vi "STAGE+mono+counter_edit16.vi"() -> ()   [LabVIEW 2017]
panel:
  out "XY Graph 2":cluster{dbl[], dbl[]}[](graph)
  out "XY Graph":cluster{dbl[], dbl[]}(graph)
  out "PROGRESS":u8(slide) max=10 step=10 scale=0.0..1.0
  in  "?":enum32{"DELAY", "COUNTER", "MONO", "PLOT"}(tab)
  out "Final time [ps]":dbl
  out "Current time [ps]":dbl
  out "Initial time [ps]":dbl
  in  "Set this as t0":bool
  in  "Axis":i32=1
  in  "Motor ON":bool
  in  "Motor OFF":bool
  out "Current Position [mm]":dbl
  out "Final Position [mm]":dbl
  in  "Data Points":i32=100
  out "Current Point":i32
  in  "Step Size [um]":i32=10
  in  "Target [mm]":dbl format="%.3f"
  in  "Move":bool
  out "Initial position [mm]":dbl
  in  "GPIB address":string="23"
  in  "Count Mode":u16(ring) items=["A,B for Preset T", "A-B for Preset T", "A+B for Preset T", "A for Preset B"]
  in  "Trigger mode":u16(ring) items=["10 MHz"=0, "Input 2"=2, "Input T"=3]
  in  "Channel A Input":u16(ring)=1 items=["10 MHz", "Input 1"]
  in  "Channel B Input":u16(ring)=2 items=["Input 1"=1, "Input 2"=2]
  in  "Number of Measurements\n to take at one point/ Number of Periods":u16=1 min=1 max=2000 step=1
  in  "Time between measurements\n at one point (s)/Dwell Time":dbl=0.002 min=0.002 max=60.0 step=0.001
  in  "gate mode (CW:0)":i16(slide) scale=0.0..2.0 scale format="%.2f"
  out "Counts":i32
  in  "Integrating time \nin 10^-7 sec":dbl=10000000.0
  in  "Discriminator Level (mV)":dbl min=-300.0 max=300.0 step=0.2
  in  "Discriminator Slope":bool
  in  "Channel":i16 min=0 max=2 step=1
  out "Grating #":dbl
  out "Blaze angle":dbl
  out "Grooves/mm":dbl
  out "Mono port":T1(ring)
  out "Time delay":u32=450000 min=1
  in  "Step size":dbl=10.0 min=0.0
  in  "Scan to":i32=4000
  in  "Scan from":i32=2600
  out "Current wavelength":dbl
  in  "?":bool
  in  "Array":dbl[](array[numeric])
  out "Numeric":i32
  out "Numeric 2":i32
  out "Timeout 2":bool
  in  "?":bool
  out "Timeout":bool
  in  "Collect Data!":bool
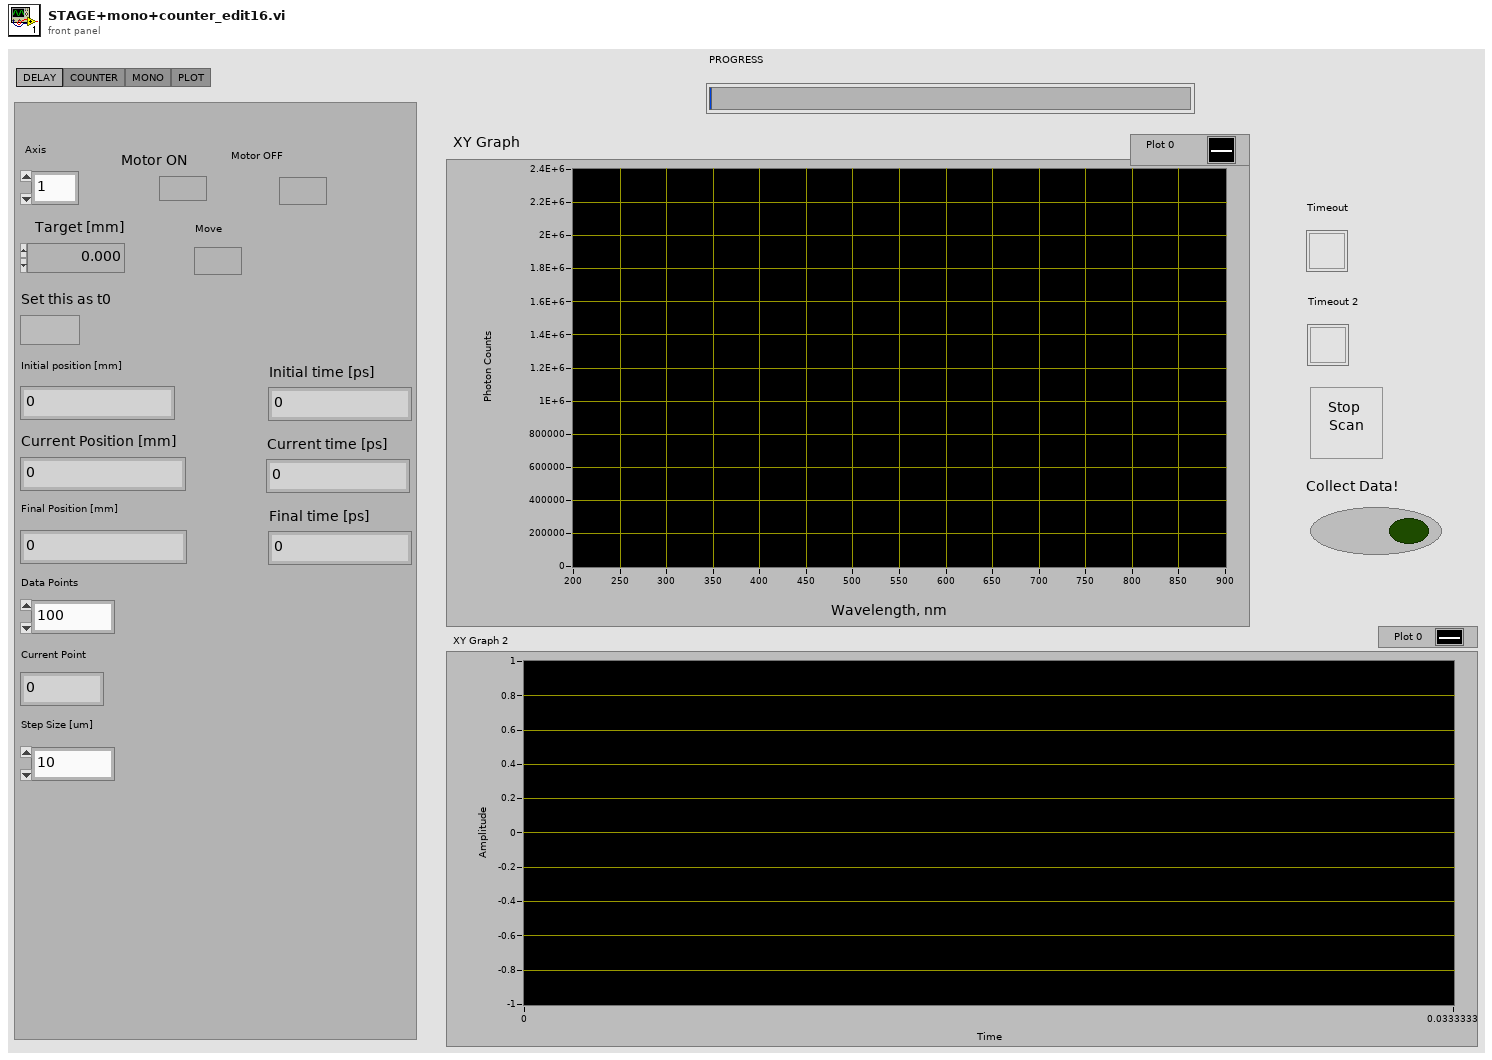
[diagram p1: front panel]
types:
  T1 = enum8{"COM 1", "COM 2", "COM 3", "COM 4", "COM 5", "COM 6", "COM 7", "COM 8", "COM 9"}
  T2 = cluster{"input XON/XOFF":bool, "input HW Handshake":bool, "input alt HW HShk":bool, "output XON/XOFF":bool, "output HW Handshake":bool, "output alt HW HShk":bool, "XOFF byte":u8, "XON byte":u8, "parity error byte":u16}
  T3 = enum16{"no parity", "odd parity", "even parity", "mark parity", "space parity"}
  T4 = cluster{"Y[0]":dbl, "Y[1]":dbl, "Y[2]":dbl, "Y[3]":dbl, "Y[4]":dbl, "Y[5]":dbl, "Y[6]":dbl, "Y[7]":dbl, "Y[8]":dbl}
  T5 = typedef "NI_Matrix.lvlib/RealMatrix.ctl" = dbl[][]
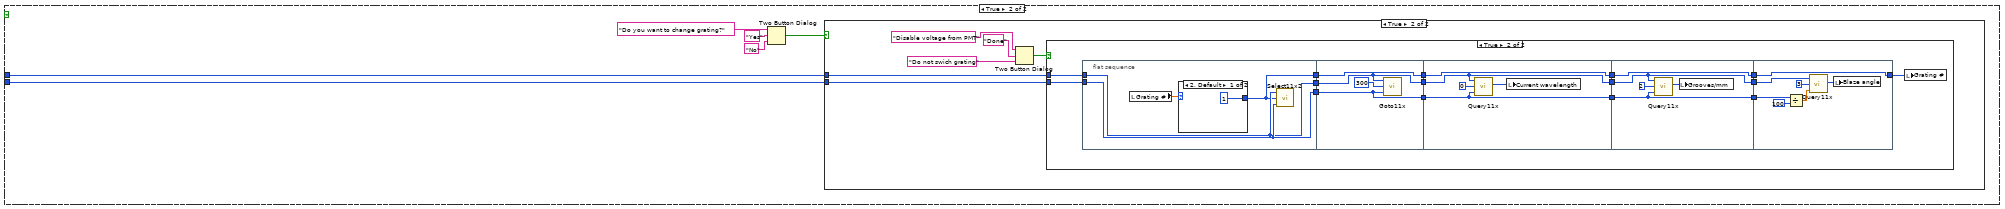
[diagram p2: hidden frame]
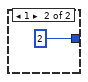
[diagram p5: hidden frame]
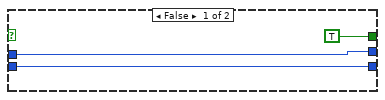
[diagram p6: hidden frame]
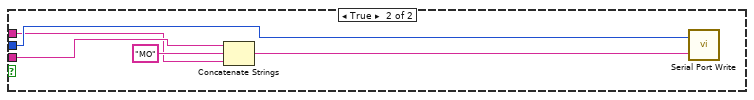
[diagram p7: hidden frame]
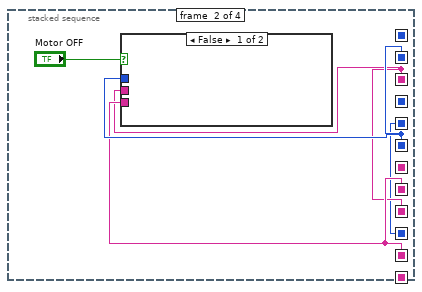
[diagram p8: hidden frame]
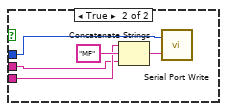
[diagram p9: hidden frame]
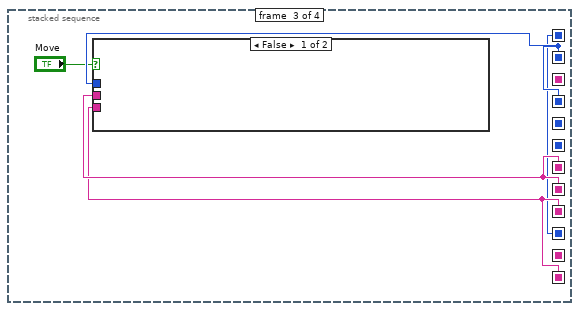
[diagram p10: hidden frame]
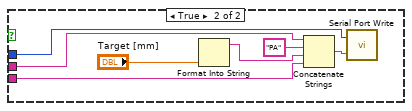
[diagram p11: hidden frame]
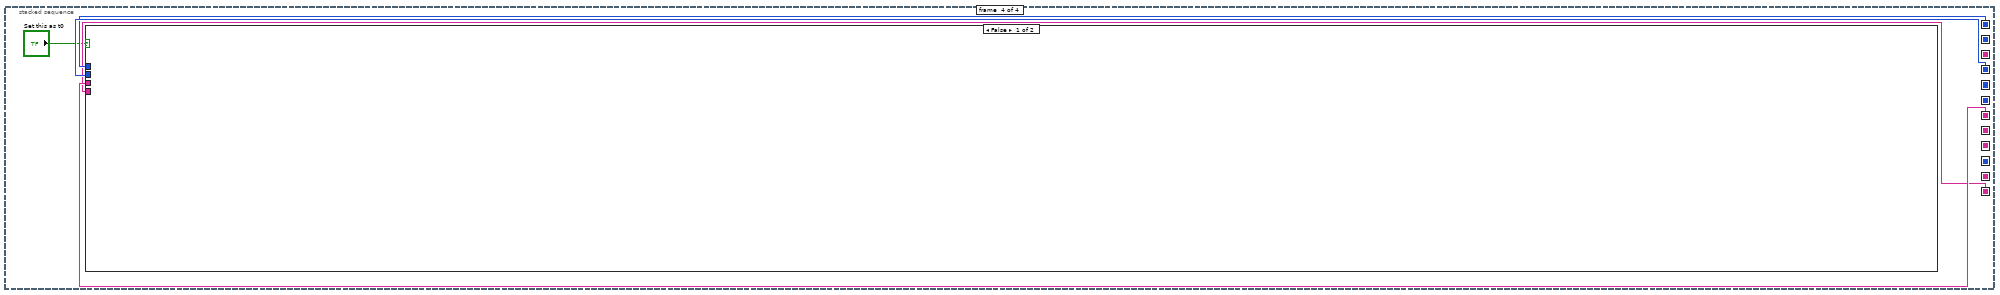
[diagram p12: hidden frame]
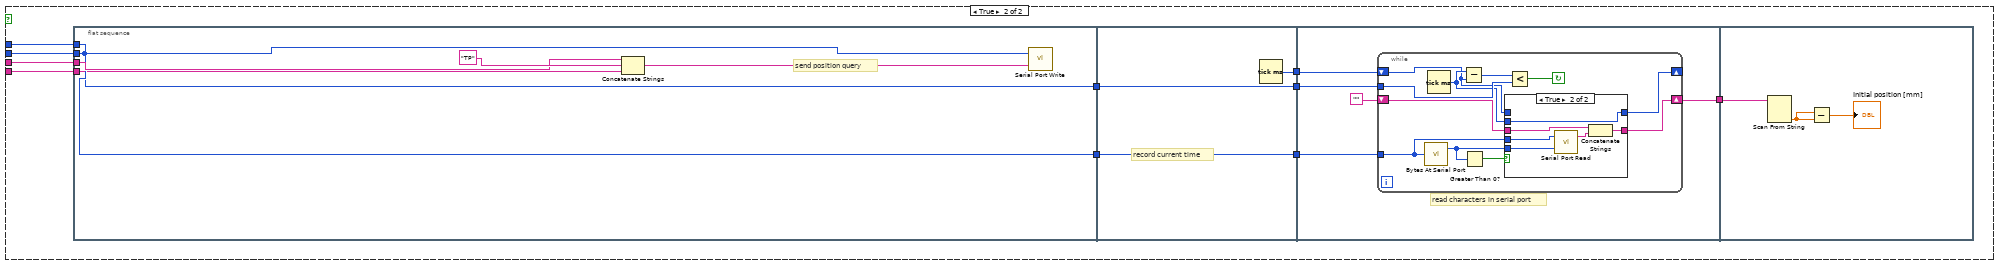
[diagram p13: hidden frame]
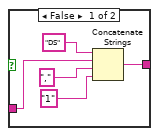
[diagram p15: hidden frame]
diagram:
  (unwired) FALSE
  w39 = u32 19200  # baud rate
  w38 = u16 8  # data bits
  w37 = enum16{"1 bit", "1.5 bits", "2 bits"}."1 bit"  # stop bits
  w41 = T3."no parity"  # parity
  w36 = 4  # 0=COM1 so n=COM(n+1)
  w40 = u16 1024  # buffer size
  n1 = flat-sequence {
    tunnel: ["Data Points"] -> w45
    tunnel: "Axis" -> [w67]
    tunnel: [w59] -> w44
    tunnel: [w67] -> w43
    tunnel: ["Step Size [um]"] -> w17
    tunnel: [w59] -> w16
    tunnel: ["Step Size [um]"] -> w15
    tunnel: ["Data Points"] -> w14
    tunnel: [w59] -> w13
    tunnel: [w58] -> w12
    tunnel: [w59] -> w10
    tunnel: [w58] -> w9
    tunnel: [w61] -> w8
    tunnel: [w51] -> w7
    tunnel: w45 -> [w151]
    tunnel: w44 -> [w150]
    tunnel: w43 -> [w149]
    tunnel: w36 -> [w145]
    tunnel: "GPIB address" -> [w144]
    tunnel: "GPIB address" -> [w143]
    tunnel: w17 -> [w131]
    tunnel: w16 -> [w129]
    tunnel: w15 -> [w128]
    tunnel: w14 -> [w126]
    tunnel: w13 -> [w121]
    tunnel: w12 -> [w120]
    tunnel: "Integrating time \nin 10^-7 sec" -> [w119]
    tunnel: w10 -> [w117]
    tunnel: w9 -> [w116]
    tunnel: w8 -> [w115]
    tunnel: w7 -> [w113]
    tunnel: w3 -> [w94]
    tunnel: w2 -> [w93]
    tunnel: w1 -> [w92]
    frame #0 {
      n2 = while {
        stop <- "Collect Data!" stop-if-true
        n3 = Multiply(x=1, y=1000) -> (x*y=w49:i32)
        n4 = Wait (ms)(milliseconds to wait=w49) -> ()  [unwired: 1 out]
      }
    }
    frame #1 {
      w52 = 1000000000000.0
      w57 = 1000
      w60 = 300000000
      w62 = 1000
      n5 = local read "Initial position [mm]"() -> (w59:dbl)
      n6 = Multiply(x="Step Size [um]", y="Data Points") -> (x*y=w66:i32)
      n7 = Divide(x=w66, y=w62) -> (x/y=w65:dbl)
      n8 = Divide(x="Step Size [um]", y=w62) -> (x/y=w61:dbl)
      n9 = Add(x=w59, y=w65) -> (x+y=w58:dbl)
      "Final Position [mm]" <- w58
      n10 = Divide(x=w59, y=w57) -> (x/y=w55:dbl)
      n11 = Divide(x=w58, y=w57) -> (x/y=w56:dbl)
      n12 = Divide(x=w55, y=w60) -> (x/y=w54:dbl)
      n13 = Divide(x=w56, y=w60) -> (x/y=w53:dbl)
      n14 = Multiply(x=w53, y=w52) -> (x*y=→"Final time [ps]":dbl)
      n15 = Multiply(x=w54, y=w52) -> (x*y=w51:dbl)
      "Initial time [ps]" <- w51
    }
    frame #2 {
      w74 = "\r\n"
      n16 = Increment(x=w126) -> (x+1=w127:i32)
      n17 = Divide(x=w131, y=1000.0) -> (x/y=w107:dbl)
      n18 = for {
        N: w127 -> [_]
        tunnel: w107 -> [w162]
        tunnel: w129 -> [w160]
        tunnel: [w153] -> w125 mode=indexing
        i -> [w161]
        # "distances"
        n19 = Multiply(x=w162, y=w161) -> (x*y=w159:dbl)
        n20 = Add(x=w160, y=w159) -> (x+y=w158:dbl)
        n21 = Divide(x=w158, y=1000) -> (x/y=w152:dbl)
        n22 = Divide(x=w152, y=300000000) -> (x/y=w155:dbl)
        n23 = Multiply(x=w155, y=1000000000000.0) -> (x*y=w153:dbl)
      }
      n24 = Multiply(x="Scan to", y=1) -> (x*y=w114:i32)
      n25 = Multiply(x=1, y="Scan from") -> (x*y=w103:i32)
      n26 = Divide(x=w107, y=1000.0) -> (x/y=w108:dbl)
      n27 = Subtract(x=w114, y=w103) -> (x-y=w138:i32)
      n28 = local read "Numeric 2"() -> (w96:i32)
      n29 = local read "Numeric"() -> (w95:i32)
      n30 = Divide(x=w138, y="Step size") -> (x/y=w137:dbl)
      n31 = Divide(x=w108, y=300000000) -> (x/y=w110:dbl)
      n32 = Multiply(x=w110, y=1000000000000.0) -> (x*y=w106:dbl)
      n33 = Build Array(w113) -> (w100:dbl[])
      n34 = Round Toward -Infinity(1:w137) -> (0:w136:dbl)
      n35 = Concatenate Strings("\r", "\n") -> (w146:string)
      n36 = Initialize Array(0, w95, w96) -> (w98:i32[][])
      n37 = Increment(x=w136) -> (x+1=w102:dbl)
      n38 = for {
        N: w151 -> [w213]
        tunnel: w150 -> [w240]
        tunnel: w128 -> [w236]
        tunnel: w149 -> [w233]
        tunnel: w146 -> [w230]
        tunnel: w145 -> [w231]
        tunnel: w144 -> [w229]
        tunnel: w93 -> [w226]
        tunnel: w94 -> [w228]
        tunnel: w143 -> [w227]
        tunnel: [w178] -> w134 mode=indexing
        tunnel: w103 -> [w221]
        tunnel: "Step size" -> [w220]
        tunnel: w136 -> [w219]
        tunnel: w121 -> [_]
        tunnel: w120 -> [_]
        tunnel: w119 -> [w218]
        tunnel: "Scan to" -> [w217]
        tunnel: "Scan from" -> [w216]
        tunnel: "Step size" -> [w187]
        tunnel: w117 -> [w208]
        tunnel: w116 -> [w206]
        tunnel: w115 -> [w209]
        tunnel: w106 -> [w196]
        shift-right: [w180] -> _
        shift-left: w100 -> [w190]
        shift-right: [w179] -> _
        shift-left: dbl[] [] ("Y") -> [w185]
        tunnel: w113 -> [w214]
        tunnel: "Scan from" -> [w188]
        tunnel: "Step size" -> [w189]
        shift-right: [w177] -> _
        shift-left: w100 -> [w183]
        shift-right: [w175] -> _
        shift-left: w98 -> [w174]
        tunnel: w94 -> [w170]
        tunnel: w93 -> [w169]
        tunnel: w92 -> [w168]
        i -> [w195]
        w207 = 1000
        w210 = 300000000
        n39 = To Time Stamp(1:w221) -> ()  [unwired: 1 out]
        n40 = property on="PROGRESS" class="Slide (strict)"("Scale.Increment"=1, "Scale.Maximum"=w213, "Scale.Minimum"=0) -> ()  [unwired: 2 in, 2 out]
        n41 = stacked-sequence {
          tunnel: w226 -> [w466]
          tunnel: w227 -> [_]
          frame #0 {
            n42 = call <vilib>:"Close Serial Driver.vi"("port number"=w466) -> ()  [unwired: 1 out]
            n43 = GPIB Misc(0:"loc 23" ("command string")) -> ()  [unwired: 1 in, 3 out]
          }
        }
        n44 = Multiply(x=w196, y=w195) -> (x*y=w215:dbl)
        n45 = Divide(x=w208, y=w207) -> (x/y=w204:dbl)
        n46 = Divide(x=w206, y=w207) -> (x/y=w203:dbl)
        n47 = Divide(x=w209, y=w207) -> (x/y=w205:dbl)
        n48 = Number To Decimal String(number=w218) -> (decimal integer string=w224:string)  [unwired: 1 in]
        n49 = Build Array(w188) -> (w192:i32[])
        n50 = Add(x=1, y=w195) -> (x+y=→"PROGRESS":i32)
        n51 = Divide(x=w236, y=1000) -> (x/y=w235:dbl)
        n52 = Divide(x=w204, y=w210) -> (x/y=w198:dbl)
        n53 = Divide(x=w203, y=w210) -> (x/y=w197:dbl)
        n54 = Divide(x=w205, y=w210) -> (x/y=w199:dbl)
        n55 = Add(x=w214, y=w215) -> (x+y=w184:dbl)
        n56 = Concatenate Strings("CP 2,", w224) -> (w222:string)
        n57 = flat-sequence {
          tunnel: w229 -> [w257]
          tunnel: w228 -> [w256]
          tunnel: w226 -> [w255]
          tunnel: w221 -> [w254]
          tunnel: w220 -> [w253]
          tunnel: w219 -> [w252]
          tunnel: w217 -> [w251]
          tunnel: w216 -> [w250]
          tunnel: w192 -> [w249]
          tunnel: dbl[] [] ("Y") -> [w248]
          tunnel: w189 -> [w247]
          tunnel: w188 -> [w246]
          tunnel: w187 -> [w245]
          tunnel: [w244] -> w186
          tunnel: w170 -> [w243]
          tunnel: w169 -> [w242]
          tunnel: w168 -> [w241]
          tunnel: w186 -> [w420]
          tunnel: w185 -> [w427]
          tunnel: [w420] -> w182
          tunnel: w181 -> [w424]
          tunnel: [w422] -> w180
          tunnel: [w421] -> w179
          tunnel: [w420] -> w178
          tunnel: w182 -> [w436]
          tunnel: [w429] -> w177
          tunnel: w176 -> [w430]
          tunnel: w174 -> [w433]
          tunnel: [w431] -> w175
          frame #0 {
            # "step size"
            n58 = while {
              tunnel: w255 -> [_]
              tunnel: w256 -> [_]
              tunnel: w257 -> [w260]
              tunnel: w254 -> [w291]
              tunnel: w253 -> [w290]
              tunnel: w252 -> [w289]
              tunnel: w251 -> [w274]
              tunnel: w250 -> [w275]
              tunnel: w245 -> [w276]
              tunnel: w247 -> [w287]
              shift-right: [w283] -> w244
              shift-left: w248 -> [w282]
              shift-right: [w277] -> _
              shift-left: w249 -> [w285]
              tunnel: w246 -> [w280]
              tunnel: w243 -> [w264]
              tunnel: w242 -> [w263]
              tunnel: w241 -> [w262]
              i -> [w288]
              stop <- w294 stop-if-true
              n59 = property on="XY Graph" class="XYGraph (strict)"("XScale.Increment"=w276, "XScale.Maximum"=w274, "XScale.Minimum"=w275) -> ()  [unwired: 2 in, 2 out]
              n60 = Multiply(x=w288, y=w290) -> (x*y=w295:dbl)
              n61 = Multiply(x=w288, y=w287) -> (x*y=w286:dbl)
              n62 = Greater Or Equal?(x=w288, y=w289) -> (x >= y?=w292:bool)
              n63 = Add(x=w286, y=w280) -> ()  [unwired: 1 out]
              n64 = Add(x=w295, y=w291) -> (x+y=w261:dbl)
              n65 = flat-sequence {
                tunnel: w260 -> [w310]
                tunnel: w261 -> [w311]
                tunnel: [w311] -> w268
                tunnel: [w297] -> w267
                tunnel: [w296] -> w266
                tunnel: [w310] -> w265
                tunnel: w264 -> [w300]
                tunnel: w263 -> [w299]
                tunnel: w262 -> [w298]
                tunnel: [w344] -> w273
                tunnel: [w343] -> w272
                tunnel: [w341] -> w271
                tunnel: w268 -> [w345]
                tunnel: w267 -> [w344]
                tunnel: w266 -> [w343]
                tunnel: w265 -> [w341]
                tunnel: w273 -> [w352]
                tunnel: w272 -> [w351]
                tunnel: w271 -> [w346]
                tunnel: [w346] -> w259
                tunnel: w259 -> [w354]
                tunnel: [w354] -> w258
                tunnel: w258 -> [w407]
                tunnel: [w407] -> w270
                tunnel: w270 -> [w408]
                tunnel: [w408] -> w269
                tunnel: [w414] -> w279
                tunnel: w269 -> [w415]
                frame #0 {
                  n66 = flat-sequence {
                    tunnel: w300 -> [w317]
                    tunnel: [w317] -> w309
                    tunnel: w299 -> [w319]
                    tunnel: [w319] -> w308
                    tunnel: w298 -> [w315]
                    tunnel: [w315] -> w307
                    tunnel: w309 -> [w323]
                    tunnel: [w323] -> w306
                    tunnel: w308 -> [w324]
                    tunnel: [w324] -> w305
                    tunnel: w307 -> [w321]
                    tunnel: [w321] -> w304
                    tunnel: w306 -> [w332]
                    tunnel: [w332] -> w303
                    tunnel: w305 -> [w329]
                    tunnel: [w329] -> w302
                    tunnel: w304 -> [w327]
                    tunnel: [w327] -> w301
                    tunnel: w303 -> [w334]
                    tunnel: w302 -> [w335]
                    tunnel: w301 -> [_]
                    tunnel: [w335] -> w297
                    tunnel: [w334] -> w296
                    frame #0 {
                      n67 = call "Query11x.vi"("port number"=w319, "QUERY"=u16 0, "time delay"=w317) -> ("timeout"=w316:bool, "STATUS MESSAGE"=w314:u16)  [unwired: 2 out]
                      n68 = local write "Timeout"(w316) -> ()
                      n69 = Divide(x=w314, y=1 ("Numeric")) -> (x/y=→"Current wavelength":dbl)
                    }
                    frame #1 {
                      n70 = call "Query11x.vi"("port number"=w324, "QUERY"=u16 2, "time delay"=w323) -> ("timeout"=w322:bool, "STATUS MESSAGE"=→"Grooves/mm":u16)  [unwired: 2 out]
                      n71 = local write "Timeout"(w322) -> ()
                    }
                    frame #2 {
                      n72 = Divide(x=w332, y=i16 100 ("device (1)")) -> (x/y=w330:dbl)
                      n73 = call "Query11x.vi"("port number"=w329, "QUERY"=u16 3, "time delay"=w330) -> ("timeout"=w328:bool, "STATUS MESSAGE"=→"Blaze angle":u16)  [unwired: 2 out]
                      n74 = local write "Timeout"(w328) -> ()
                    }
                    frame #3 {
                      n75 = Divide(x=w334, y=i16 100 ("device (1)")) -> (x/y=w338:dbl)
                      n76 = call "Query11x.vi"("port number"=w335, "QUERY"=u16 4, "time delay"=w338) -> ("timeout"=w337:bool, "STATUS MESSAGE"=→"Grating #":u16)  [unwired: 2 out]
                      n77 = local write "Timeout"(w337) -> ()
                    }
                  }
                }
                frame #1 {
                  n78 = call "Goto11x.vi"("time delay"=w343, "WAVELENGTH"=w345, "port number"=w344) -> ("timeout"=w342:bool)  [unwired: 2 out]
                  n79 = local write "Timeout 2"(w342) -> ()
                }
                frame #2 {
                  # "set counter time in 10^-7 seconds in CW"
                  n80 = call "Query11x.vi"("port number"=w352, "QUERY"=0, "time delay"=w351) -> ("timeout"=w350:bool, "STATUS MESSAGE"=w349:u16)  [unwired: 2 out]
                  n81 = local write "Timeout 2"(w350) -> ()
                  n82 = Divide(x=w349, y=1) -> (x/y=w348:dbl)
                  n83 = local write "Current wavelength"(w348) -> ()
                }
                frame #3 {
                  # "Configures discriminator."
                  n84 = flat-sequence {
                    tunnel: w354 -> [w364]
                    tunnel: [w364] -> w363
                    tunnel: [w371] -> w362
                    tunnel: [w369] -> w361
                    tunnel: "Discriminator Slope" -> [w370]
                    tunnel: w363 -> [w369]
                    tunnel: w355 -> [w368]
                    tunnel: w362 -> [w390]
                    tunnel: [w391] -> w360
                    tunnel: w361 -> [w389]
                    tunnel: [w389] -> w359
                    tunnel: w355 -> [w387]
                    tunnel: w360 -> [w403]
                    tunnel: w359 -> [w402]
                    tunnel: "Discriminator Level (mV)" -> [w397]
                    tunnel: w355 -> [w396]
                    frame #0 {
                      # "Flush I/O buffers."
                      n85 = for {
                        N: 5 -> [_]
                        tunnel: w364 -> [w366]
                        n86 = GPIB Write(0:w366, 1:"\r") -> ()  [unwired: 3 in, 2 out]
                      }
                    }
                    frame #1 {
                      # "Set discriminator slope."
                      n87 = case shown="True" w370 {
                        tunnel: [w377 w382] -> w372
                        tunnel: w368 -> [w376 w381]
                        frame False {
                          n88 = Concatenate Strings("DS", w376, ",", "1") -> (w377:string)
                        }
                        frame True {
                          n89 = Concatenate Strings("DS", w381, ",", "0") -> (w382:string)
                        }
                      }
                      n90 = GPIB Write(0:w369, 1:w372, 2:5) -> (6:w371:errorcluster)  [unwired: 2 in, 1 out]
                    }
                    frame #2 {
                      # "Set discriminator mode to fixed."
                      n91 = Concatenate Strings("DM", w387, ",", "0") -> (w386:string)
                      n92 = GPIB Write(0:w389, 1:w386, 2:5, 3:w390) -> (6:w391:errorcluster)  [unwired: 1 in, 1 out]
                    }
                    frame #3 {
                      # "Set discriminator level.\nMust be between +300 and -300 mV."
                      n93 = Divide(x=w397, y=1000.0) -> (x/y=w405:dbl)
                      n94 = Number To Fractional String(number=w405, precision (6)=i16 4) -> (F-format string=w394:string)  [unwired: 2 in]
                      n95 = Concatenate Strings("DL", w396, ",", w394) -> (w401:string)
                      n96 = GPIB Write(0:w402, 1:w401, 2:5, 3:w403) -> (6:w398:errorcluster)  [unwired: 1 in, 1 out]
                      n97 = call <vilib>:"General Error Handler.vi"("type of dialog (OK msg:1)"=1, "error in (no error)"=w398) -> ()  [unwired: 9 in, 5 out]
                    }
                  }
                  n98 = Number To Decimal String(number="Channel") -> (decimal integer string=w355:string)  [unwired: 1 in]
                }
                frame #4 {
                  n99 = call "Start.vi"("GPIB Address"=w407) -> ()  [unwired: 9 in]
                }
                frame #5 {
                  # "Wait for Scan to Finish"
                  n100 = for {
                    N: 1 -> [_]
                    tunnel: w408 -> [w410]
                    n101 = while {
                      tunnel: w410 -> [w411]
                      stop <- w413 stop-if-true
                      n102 = call "ScanDone.vi"("Wait (ms)"=1000, "GPIB Address"=w411) -> ("Scan Finished?"=w413:bool)
                    }
                  }
                }
                frame #6 {
                  n103 = call "Read Data.vi"("Channel Number"=0, "GPIB Address"=w415, "Number of Datapoints"=1) -> ("Data"=w416:i32[])
                  n104 = Index Array(array=w416, index=0) -> (element=w414:i32)
                  "Counts" <- w414
                }
              }
              n105 = Or(x="?", y=w292) -> (x .or. y?=w294:bool)
              n106 = Build Array (concatenate)(w285, w261) -> (w284:dbl[])
              n107 = Build Array (concatenate)(w282, w279) -> (w281:dbl[])
              n108 = Bundle(w284, w281) -> (w278:cluster{dbl[], dbl[]})  [unwired: 1 in]
              "XY Graph" <- w278
              n109 = Unbundle(w278) -> (w277:dbl[], w283:dbl[])
            }
          }
          frame #1 {
            n110 = Array To Cluster(array=w420) -> (cluster=w428:T4)
            n111 = Unbundle By Name(w428) -> ("Y[5]"=w426:dbl)  [unwired: 10 out]
            n112 = Build Array (concatenate)(w427, w426) -> (w425:dbl[])
            n113 = Bundle(w424, w425) -> (w423:cluster{dbl[], dbl[]})  [unwired: 1 in]
            n114 = Unbundle(w423) -> (w422:dbl[], w421:dbl[])
          }
          frame #2 {
            n115 = Array Size(array="Array") -> (size(s)=w434:i32)
            n116 = flat-sequence {
              tunnel: w436 -> [w441]
              tunnel: "Array" -> [w440]
              tunnel: w434 -> [w439]
              tunnel: [w437] -> w432
              tunnel: w433 -> [w458]
              tunnel: w432 -> [w457]
              tunnel: [w455] -> w431
              tunnel: w430 -> [w454]
              tunnel: [w453] -> w429
              frame #0 {
                n117 = for {
                  N: w439 -> [w443]
                  tunnel: w440 -> [w451]
                  tunnel: w441 -> [w445]
                  tunnel: [w442] -> w438
                  i -> [w450]
                  n118 = local read "Scan from"() -> (w448:i32)
                  n119 = Index Array(array=w451, index=w450) -> (element=w449:dbl)
                  n120 = local read "Step size"() -> (w446:dbl)
                  n121 = Subtract(x=w449, y=w448) -> (x-y=w447:dbl)
                  n122 = Divide(x=w447, y=w446) -> (x/y=w444:dbl)
                  n123 = Index Array(array=w445, index=w444) -> (element=w442:dbl)
                  "Numeric" <- w443
                }
                n124 = Build Array(w438) -> (w437:dbl[])
              }
              frame #1 {
                n125 = local read "Numeric"() -> (w456:i32)
                n126 = Build Array (concatenate)(w458, w457) -> (w455:dbl[][])
                n127 = for {
                  N: w456 -> [_]
                  tunnel: w455 -> [w464]
                  tunnel: w454 -> [w462]
                  tunnel: [w461] -> w453
                  tunnel: [w459] -> w452 mode=indexing
                  i -> [w463]
                  n128 = Index Array(array=w464, index (row)=w463) -> (element=w460:dbl[])  [unwired: 1 in]
                  n129 = Bundle(w462, w460) -> (w459:cluster{dbl[], dbl[]})  [unwired: 1 in]
                  n130 = Unbundle(w459) -> (w461:dbl[])  [unwired: 1 out]
                }
                "XY Graph 2" <- w452
              }
            }
          }
        }
        n131 = Multiply(x=w235, y=w195) -> (x*y=w239:dbl)
        n132 = Multiply(x=w198, y=1000000000000.0) -> (x*y=w172:dbl)
        n133 = Multiply(x=w197, y=1000000000000.0) -> (x*y=w171:dbl)
        n134 = Multiply(x=w199, y=1000000000000.0) -> (x*y=w173:dbl)
        n135 = Build Array (concatenate)(w190, w184) -> (w181:dbl[])
        n136 = Build Array (concatenate)(w183, w184) -> (w176:dbl[])
        n137 = property on="XY Graph 2" class="XYGraph (strict)"("XScale.Increment"=w173, "XScale.Maximum"=w171, "XScale.Minimum"=w172) -> ()  [unwired: 2 in, 2 out]
        n138 = Add(x=w240, y=w239) -> (x+y=w238:dbl)
        n139 = Format Into String(w233) -> (resulting string=w232:string)  [unwired: 3 in, 1 out]
        n140 = GPIB Write(0:w229, 1:w222, 2:i16 5 ("mode (0)")) -> ()  [unwired: 2 in, 2 out]
        n141 = flat-sequence {
          tunnel: w238 -> [w469]
          tunnel: [w469] -> w234
          tunnel: w230 -> [w471]
          tunnel: w232 -> [w470]
          tunnel: w231 -> [w467]
          tunnel: w234 -> [w480]
          frame #0 {
            n142 = Format Into String(w469) -> (resulting string=w468:string)  [unwired: 3 in, 1 out]
            n143 = Wait (ms)(milliseconds to wait=u32 100) -> ()  [unwired: 1 out]
            n144 = Concatenate Strings(w470, "PA" ("Substring"), w468, w471) -> (w473:string)
            n145 = call <vilib>:"Serial Port Write.vi"("string to write"=w473, "port number"=w467) -> ()  [unwired: 1 out]
          }
          frame #1 {
            n146 = Divide(x=w480, y=1000) -> (x/y=w478:dbl)
            n147 = Wait (ms)(milliseconds to wait=u32 1000) -> ()  [unwired: 1 out]
            n148 = Divide(x=w478, y=300000000) -> (x/y=w477:dbl)
            n149 = Multiply(x=w477, y=1000000000000.0) -> (x*y=→"Current time [ps]":dbl)
            "Current Position [mm]" <- w480
          }
        }
        "Current Point" <- w195
        "Numeric 2" <- w213
      }
      n150 = for {
        N: w102 -> [_]
        tunnel: "Step size" -> [w167]
        tunnel: w103 -> [w165]
        tunnel: [w163] -> w101 mode=indexing
        i -> [w166]
        # "wavelengths"
        n151 = Multiply(x=w167, y=w166) -> (x*y=w164:dbl)
        n152 = Add(x=w165, y=w164) -> (x+y=w163:dbl)
      }
      n153 = Build Array (concatenate)(0, w125) -> (w68:dbl[])
      n154 = Build Array(w101) -> (w135:dbl[][])
      n155 = local read "Integrating time \nin 10^-7 sec"() -> (w72:dbl)
      n156 = Transpose Matrix(1:w134) -> (0:w132:dbl[][])
      n157 = Transpose Matrix(1:w135) -> (0:w133:dbl[][])
      n158 = Build Array (concatenate)(w133, w132) -> (w69:T5)
      n159 = Insert Into Array(array=w69, index (row)=0, new element=w68) -> (w122:T5)  [unwired: 1 in]
      n160 = local read "Blaze angle"() -> (w91:dbl)
      n161 = local read "Grating #"() -> (w90:dbl)
      n162 = Multiply(x=w72, y=1e-07) -> (x*y=w71:dbl)
      n163 = Get Date/Time In Seconds() -> (seconds since 1Jan1904=w84:timestamp)
      n164 = Array To Spreadsheet String(delimiter (Tab)=",", array=w122, 3:"%f" ("format string")) -> (spreadsheet string=w73:string)
      n165 = Number To Decimal String(number=w91) -> (decimal integer string=w75:string)  [unwired: 1 in]
      n166 = Format Date/Time String(time format string (%c)="%Y-%b-%d %H:%M:%S", seconds (now)=w84) -> (date/time string=w85:string)  [unwired: 1 in]
      n167 = Number To Decimal String(number=w71) -> (decimal integer string=w86:string)  [unwired: 1 in]
      n168 = Number To Decimal String(number=w90) -> (decimal integer string=w87:string)  [unwired: 1 in]
      n169 = call <vilib>:"Space Constant.vi"() -> ("String"=w88:string)
      n170 = Concatenate Strings(w74, "Data was taken on ", w85, w74, "Integration Time is ", w86, w88, "s", w74, "Monochromator gratng # ", w87, "; ", "blazed for ", w75, w88, "nm", w74, w74, w74, w73) -> (w89:string)
      n171 = Write to Text File(text=w89) -> ()  [unwired: 3 in, 3 out]
    }
  }
  n172 = flat-sequence {
    tunnel: [w484] -> w30
    tunnel: [w483] -> w29
    frame #0 {
      n173 = call "CM Com Read ini.vi"() -> ("Mono port"=w483:T1, "time delay1"=w484:u32)  [unwired: 7 in]
    }
  }
  n174 = call <vilib>:"Serial Port Init.vi"("flow control etc."=T2 {"input XON/XOFF"=FALSE, "input HW Handshake"=FALSE, "input alt HW HShk"=FALSE, "output XON/XOFF"=FALSE, "output HW Handshake"=FALSE, "output alt HW HShk"=FALSE, "XOFF byte"=13, "XON byte"=11, "parity error byte"=0}, "parity"=w41, "buffer size"=w40, "stop bits"=w37, "data bits"=w38, "baud rate"=w39, "port number"=w36) -> ("error code"=w35:i32)
  n175 = call "CM Serial Port Setup.vi"("COM port"=w29, "time delay"=w30) -> ("time delay1"=w25:u32, "DK port Out"=w26:T1, "error code"=w28:i32)  [unwired: 7 in]
  n176 = Equal To 0?(x=w28) -> (x = 0?=w27:bool)
  n177 = Concatenate Strings("\r", "\n") -> (w31:string)
  n178 = while {
    tunnel: w36 -> [w487]
    tunnel: w31 -> [w488]
    tunnel: w35 -> [_]
    tunnel: "Axis" -> [w485]
    stop <- TRUE continue-if-true
    w486 = u32 200  # timeout
    n179 = Format Into String(w485) -> (resulting string=w489:string)  [unwired: 3 in, 1 out]
    n180 = stacked-sequence {
      seq-local: [w494 _ _ _] -> [_ w505 _ _]
      seq-local: [w493 _ _ _] -> [_ w504 _ _]
      seq-local: [w495 _ _ _] -> [_ w506 _ _]
      seq-local: [w492 _ _ _] -> [_ w502 _ _]
      seq-local: [_ w505 _ _] -> [_ _ w515 _]
      seq-local: [_ w504 _ _] -> [_ _ w514 _]
      seq-local: [_ w506 _ _] -> [_ _ w516 _]
      seq-local: [_ w502 _ _] -> [_ _ w512 _]
      seq-local: [_ _ w515 _] -> [_ _ _ w528]
      seq-local: [_ _ w514 _] -> [_ _ _ w525]
      seq-local: [_ _ w516 _] -> [_ _ _ w527]
      seq-local: [_ _ w512 _] -> [_ _ _ w526]
      tunnel: w489 -> [w494 _ _ _]
      tunnel: w488 -> [w493 _ _ _]
      tunnel: w487 -> [w495 _ _ _]
      tunnel: w486 -> [w492 _ _ _]
      frame #0 {
        n181 = case shown="False" "Motor ON" {
          tunnel: w495 -> [_ w501]
          tunnel: w494 -> [_ w498]
          tunnel: w493 -> [_ w497]
          frame False {
          }
          frame True {
            n182 = Concatenate Strings(w498, "MO" ("Substring"), w497) -> (w499:string)
            n183 = call <vilib>:"Serial Port Write.vi"("string to write"=w499, "port number"=w501) -> ()  [unwired: 1 out]
          }
        }
      }
      frame #1 {
        n184 = case shown="False" "Motor OFF" {
          tunnel: w506 -> [_ w511]
          tunnel: w505 -> [_ w508]
          tunnel: w504 -> [_ w507]
          frame False {
          }
          frame True {
            n185 = Concatenate Strings(w508, "MF" ("Substring"), w507) -> (w509:string)
            n186 = call <vilib>:"Serial Port Write.vi"("string to write"=w509, "port number"=w511) -> ()  [unwired: 1 out]
          }
        }
      }
      frame #2 {
        n187 = case shown="False" "Move" {
          tunnel: w516 -> [_ w523]
          tunnel: w515 -> [_ w520]
          tunnel: w514 -> [_ w519]
          frame False {
          }
          frame True {
            n188 = Format Into String("Target [mm]") -> (resulting string=w517:string)  [unwired: 3 in, 1 out]
            n189 = Concatenate Strings(w520, "PA" ("Substring"), w517, w519) -> (w521:string)
            n190 = call <vilib>:"Serial Port Write.vi"("string to write"=w521, "port number"=w523) -> ()  [unwired: 1 out]
          }
        }
      }
      frame #3 {
        n191 = case shown="False" "Set this as t0" {
          tunnel: w528 -> [_ w538]
          tunnel: w527 -> [_ w537]
          tunnel: w526 -> [_ w536]
          tunnel: w525 -> [_ w535]
          frame False {
          }
          frame True {
            n192 = flat-sequence {
              tunnel: w538 -> [w542]
              tunnel: w537 -> [w541]
              tunnel: [w541] -> w534
              tunnel: w536 -> [w539]
              tunnel: [w539] -> w533
              tunnel: w535 -> [w540]
              tunnel: w534 -> [w546]
              tunnel: [w546] -> w532
              tunnel: w533 -> [w545]
              tunnel: [w545] -> w531
              tunnel: [w547] -> w530
              tunnel: w532 -> [w552]
              tunnel: w531 -> [w550]
              tunnel: w530 -> [w549]
              tunnel: [w548] -> w529
              tunnel: w529 -> [w574]
              frame #0 {
                # "send position query"
                n193 = Concatenate Strings(w542, "TP" ("Substring"), w540) -> (w543:string)
                n194 = call <vilib>:"Serial Port Write.vi"("string to write"=w543, "port number"=w541) -> ()  [unwired: 1 out]
              }
              frame #1 {
                # "record current time"
                n195 = Tick Count (ms)() -> (millisecond timer value=w547:u32)
              }
              frame #2 {
                # "read characters in serial port"
                n196 = while {
                  shift-left: w549 -> [w553]
                  shift-right: [w554] -> _
                  tunnel: w550 -> [w557]
                  shift-left: "" -> [w560]
                  shift-right: [w559] -> w548
                  tunnel: w552 -> [w561]
                  stop <- w556 continue-if-true
                  n197 = call <vilib>:"Bytes At Serial Port.vi"("port number"=w561) -> ("byte count"=w562:u32)  [unwired: 1 out]
                  n198 = Tick Count (ms)() -> (millisecond timer value=w555:u32)
                  n199 = Subtract(x=w555, y=w553) -> (x-y=w558:u32)
                  n200 = Greater Than 0?(x=w562) -> (x > 0?=w563:bool)
                  n201 = case shown="True" w563 {
                    tunnel: w562 -> [_ w571]
                    tunnel: w561 -> [_ w570]
                    tunnel: w560 -> [w565 w568]
                    tunnel: [w565 w567] -> w559
                    tunnel: [w564 w566] -> w554
                    tunnel: w555 -> [_ w566]
                    tunnel: w553 -> [w564 _]
                    frame False {
                    }
                    frame True {
                      n202 = call <vilib>:"Serial Port Read.vi"("requested byte count"=w571, "port number"=w570) -> ("string read"=w569:string)  [unwired: 1 out]
                      n203 = Concatenate Strings(w568, w569) -> (w567:string)
                    }
                  }
                  n204 = Less?(x=w558, y=w557) -> (x < y?=w556:bool)
                }
              }
              frame #3 {
                n205 = Scan From String(input string=w574) -> (output 1=w572:dbl)  [unwired: 4 in, 3 out]
                n206 = Subtract(x=w572, y=w572) -> (x-y=→"Initial position [mm]":dbl)
              }
            }
          }
        }
      }
    }
    n207 = Wait Until Next ms Multiple(millisecond multiple=u32 50) -> ()  [unwired: 1 out]
  }
  n208 = case shown="True" w27 {
    tunnel: w26 -> [w577 w580]
    tunnel: w25 -> [w576 w579]
    tunnel: [w577 w580] -> w2
    tunnel: [w576 w579] -> w3
    tunnel: [TRUE FALSE] -> w1
    frame False {
    }
    frame True {
      n209 = call "CM Com Write ini.vi"("time delay1"=w580, "Mono port"=w579) -> ()  [unwired: 7 in]
      n210 = local write "Mono port"(w580) -> ()
      n211 = local write "Time delay"(w579) -> ()
    }
  }
  n212 = call "Configure.vi"("Dwell Time (s)"="Time between measurements\n at one point (s)/Dwell Time", "Channel T Input"="Trigger mode", "Channel B Input"="Channel B Input", "Channel A Input"="Channel A Input", "Integrating time, 10^-7 sec"="Integrating time \nin 10^-7 sec", "gate mode (CW:0)"="gate mode (CW:0)", "Scan End Mode"=FALSE, "Number of Periods"="Number of Measurements\n to take at one point/ Number of Periods", "Count Mode"="Count Mode", "GPIB Address"="GPIB address") -> ()
  n213 = case shown="False" "?" {
    tunnel: w3 -> [_ w582]
    tunnel: w2 -> [_ w581]
    frame False {
    }
    frame True {
      n214 = Two Button Dialog(message="Do you want to change grating?", 1:"No" ("F button name (\"Cancel\")"), 2:"Yes" ("T button name (\"OK\")")) -> (T button?=w583:bool)
      n215 = case shown="True" w583 {
        tunnel: w582 -> [_ w588]
        tunnel: w581 -> [_ w587]
        frame False {
        }
        frame True {
          n216 = Two Button Dialog(message="Disable voltage from PMT", 1:"Do not swich grating" ("F button name (\"Cancel\")"), 2:"Done" ("T button name (\"OK\")")) -> (T button?=w589:bool)
          n217 = case shown="True" w589 {
            tunnel: w588 -> [_ w607]
            tunnel: w587 -> [_ w606]
            frame False {
            }
            frame True {
              n218 = flat-sequence {
                tunnel: w607 -> [w611]
                tunnel: [w611] -> w604
                tunnel: w606 -> [w610]
                tunnel: [w610] -> w603
                tunnel: [w608] -> w602
                tunnel: w604 -> [w615]
                tunnel: [w615] -> w601
                tunnel: w603 -> [w616]
                tunnel: [w616] -> w600
                tunnel: w602 -> [w614]
                tunnel: [w614] -> w599
                tunnel: w601 -> [w622]
                tunnel: [w622] -> w598
                tunnel: w600 -> [w621]
                tunnel: [w621] -> w597
                tunnel: w599 -> [w619]
                tunnel: [w619] -> w596
                tunnel: w598 -> [w625]
                tunnel: [w625] -> w595
                tunnel: w597 -> [w626]
                tunnel: [w626] -> w594
                tunnel: w596 -> [w624]
                tunnel: [w624] -> w593
                tunnel: w595 -> [w630]
                tunnel: w594 -> [w631]
                tunnel: [w629] -> w605
                tunnel: w593 -> [w629]
                frame #0 {
                  n219 = local read "Grating #"() -> (w609:dbl)
                  n220 = case shown="2, Default" w609 {
                    tunnel: [1 2] -> w608
                    frame 2, Default {
                    }
                    frame 1 {
                    }
                  }
                  n221 = call "Select11x2.vi"("time delay"=w611, "NEW GRT?"=w608, "port number"=w610) -> ()  [unwired: 3 out]
                }
                frame #1 {
                  n222 = call "Goto11x.vi"("time delay"=w615, "WAVELENGTH"=u16 300, "port number"=w616) -> ()  [unwired: 3 out]
                }
                frame #2 {
                  n223 = call "Query11x.vi"("port number"=w621, "QUERY"=u16 0, "time delay"=w622) -> ("STATUS MESSAGE"=w618:u16)  [unwired: 3 out]
                  n224 = local write "Current wavelength"(w618) -> ()
                }
                frame #3 {
                  n225 = call "Query11x.vi"("port number"=w626, "QUERY"=u16 2, "time delay"=w625) -> ("STATUS MESSAGE"=w623:u16)  [unwired: 3 out]
                  n226 = local write "Grooves/mm"(w623) -> ()
                }
                frame #4 {
                  n227 = Divide(x=w630, y=i16 100 ("device (1)")) -> (x/y=w632:dbl)
                  n228 = call "Query11x.vi"("port number"=w631, "QUERY"=u16 3, "time delay"=w632) -> ("STATUS MESSAGE"=w628:u16)  [unwired: 3 out]
                  n229 = local write "Blaze angle"(w628) -> ()
                }
              }
              n230 = local write "Grating #"(w605) -> ()
            }
          }
        }
      }
    }
  }
  "Mono port" <- w29
  "Time delay" <- w30
